vi "ApplyLayoutToObject.vi"(5 "scaling settings":T1={"scaling factor"={"horizontal"=1.0, "vertical"=1.0}, "scale text"=FALSE} {"scaling factor"."vertical" min=0.0; "scaling factor"."horizontal" min=0.0}, 7 "properties to ignore":variant, 8 "error in (no error)":errorcluster, 10 "GObj Refnum":refnum<vi>, 11 "NumericWithScale Control Layout in":refnum<class "NumericWithScale Control Layout.lvclass">) -> (0 "error out":errorcluster, 3 "NumericWithScale Control Layout out":refnum<class "NumericWithScale Control Layout.lvclass">)   [LabVIEW 2012, in "NI_SE_Front Panel Layout.lvlib" / "NumericWithScale Control Layout.lvclass"]
doc: "Apply layout information to the GObj Refnum."
uses:
  NumericWithScale Control Layout.lvclass
  Scaling Factor_Options.ctl
  XY Scaling Factor.ctl
  Control Layout/Control Layout.lvclass
  NumericWithScale Control Layout.lvclass/NumericWithScale Control Layout.ctl
  Object Layout/Object Layout.lvclass/Object Layout.ctl
  Object Layout/Get UID.vi
  Object Layout/Get Unique Name.vi
  Convert UID To String.vi
  NI_SE_Front Panel Layout.lvlib
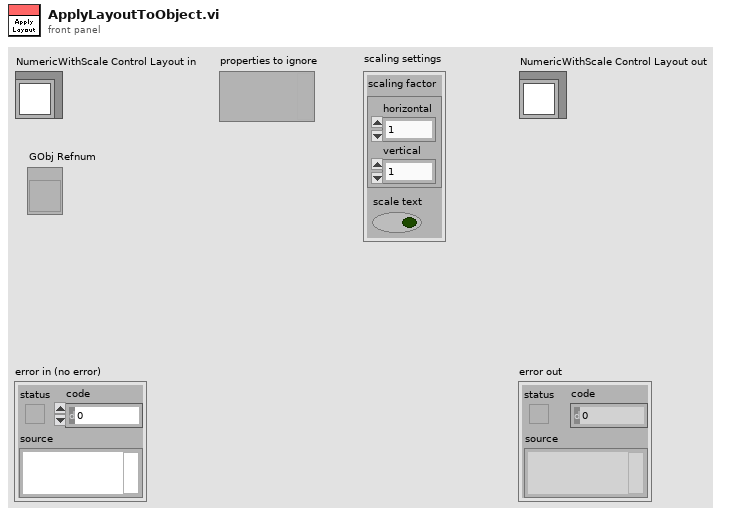
[diagram p1: front panel]
types:
  T1 = typedef "NI_SE_Front Panel Layout.lvlib/Scaling Factor_Options.ctl" = cluster{"scaling factor":T2, "scale text":bool}
  T2 = typedef "NI_SE_Front Panel Layout.lvlib/XY Scaling Factor.ctl" = cluster{"horizontal":dbl, "vertical":dbl}
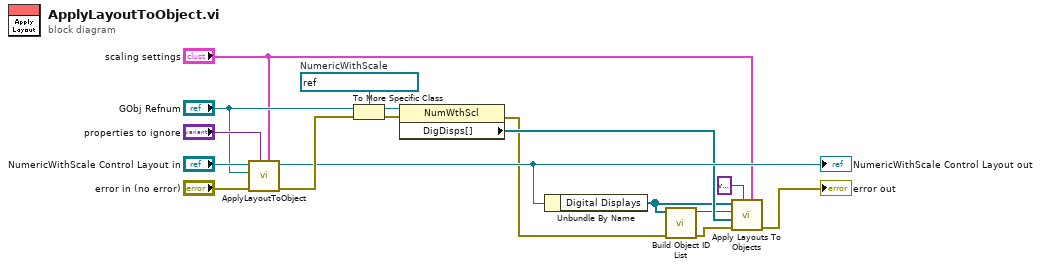
[diagram p0: block diagram]
diagram:
  w12 = refnum<vi> refnum  # NumericWithScale
  n1 = call-parent "ApplyLayoutToObject.vi"("scaling settings"="scaling settings", "properties to ignore"="properties to ignore", "error in (no error)"="error in (no error)", "GObj Refnum"="GObj Refnum", "Control Layout in"="NumericWithScale Control Layout in") -> ("error out"=w14:errorcluster, "Control Layout out"=w9:refnum<class "NumericWithScale Control Layout.lvclass">)  [unwired: 5 in]
  "NumericWithScale Control Layout out" <- w9
  n2 = To More Specific Class(target class=w12, reference="GObj Refnum", error in=w14) -> (specific class reference=w11:refnum<vi>, error out=w10:errorcluster)
  n3 = property class="NumWthScl"(reference=w11, error in=w10) -> (error out=w2:errorcluster, "DigDisps[]"=w7:refnum<vi>[])  [unwired: 1 out]
  n4 = Unbundle By Name(w9) -> ("Digital Displays"=w6:refnum<class "Digital Control Layout.lvclass">[])
  n5 = call "Build Object ID List.vi"("error in"=w2, "object layouts"=w6) -> ("error out"=w3:errorcluster, "object ID list"=w5:variant)  [unwired: 8 in]
  n6 = call "Apply Layouts To Objects.vi"("scaling settings"="scaling settings", "properties to ignore"=variant, "error in"=w3, "GObj refnums"=w7, "object ID list in"=w5, "object layouts in"=w6) -> ("error out"=→"error out":errorcluster)  [unwired: 3 in, 2 out]
